vi "Set Thermostat Mode.vi"(7 "Use Cached Data?":bool, 8 "Error In":errorcluster, 9 "Thermostat Mode":T1, 10 "Device Name":string, 11 "Nest Config":T2) -> (0 "Error Out":errorcluster, 3 "Nest Config":T2)   [LabVIEW 2013, in "LMH-Nest.lvlib"]
doc: "Set the mode of the specified Nest device (Heat, Cool, Heat/Cool)."
uses:
  LMH-Nest.lvlib
  Private/Type Defs/Nest Config.ctl
  <vilib>/httpClient/ClientHandle.ctl
  Private/Type Defs/Session Data.ctl
  Private/Type Defs/Thermostat Mode.ctl
  <vilib>/httpClient/LabVIEWHTTPClient.lvlib
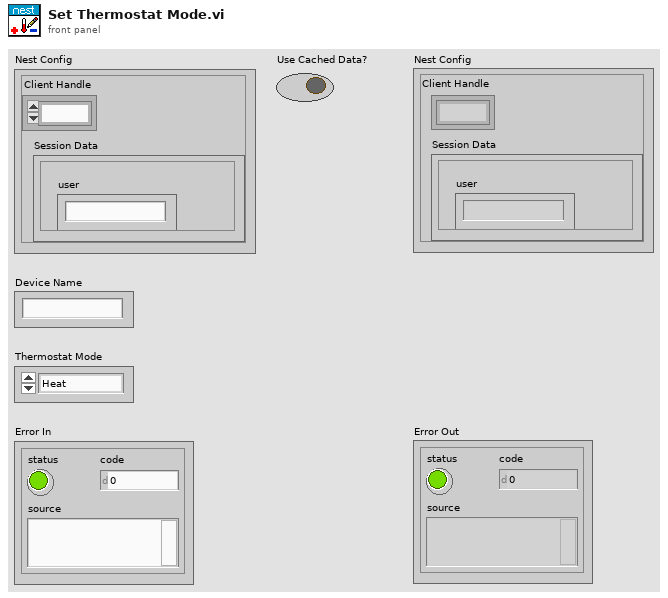
[diagram p1: front panel]
types:
  T1 = typedef "LMH-Nest.lvlib/Thermostat Mode.ctl" = enum16{"Heat", "Cool", "Heat / Cool"}
  T2 = typedef "LMH-Nest.lvlib/Nest Config.ctl" = cluster{"Client Handle":T3, "Session Data":T4}
  T3 = typedef "LabVIEWHTTPClient.lvlib/ClientHandle.ctl" = refnum<k1>
  T4 = typedef "LMH-Nest.lvlib/Session Data.ctl" = cluster{"is_superuser":bool, "is_staff":bool, "urls":cluster{"transport_url":string, "rubyapi_url":string, "weather_url":string, "log_upload_url":string, "support_url":string}, "limits":cluster{"thermostats_per_structure":u32, "structures":u32, "thermostats":u32, "smoke_detectors":u32, "smoke_detectors_per_structure":u32}, "access_token":string, "userid":string, "expires_in":string, "email":string, "user":string, "language":string}
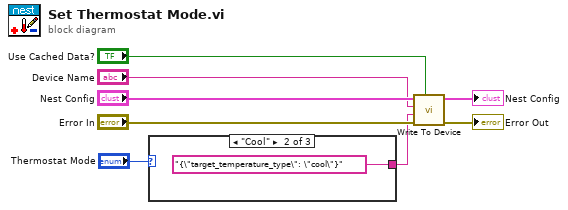
[diagram p0: block diagram]
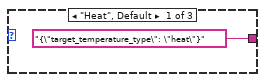
[diagram p2: hidden frame]
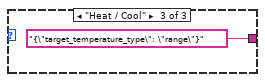
[diagram p3: hidden frame]
diagram:
  n1 = case shown="\"Cool\"" "Thermostat Mode" {
    tunnel: ["{\"target_temperature_type\": \"heat\"}" ("format string") "{\"target_temperature_type\": \"cool\"}" ("format string") "{\"target_temperature_type\": \"range\"}" ("format string")] -> w1
    frame "Heat", Default {
    }
    frame "Cool" {
    }
    frame "Heat / Cool" {
    }
  }
  n2 = call "Write To Device.vi"("Use Cached Data?"="Use Cached Data?", "Error In"="Error In", "Post Data"=w1, "Device Name"="Device Name", "Nest Config"="Nest Config") -> ("Error Out"=→"Error Out":errorcluster, "Nest Config"=→"Nest Config":T2)  [unwired: 5 in]
